vi "ziExample-UHFLI-Module-AWG.vi"() -> ()   [LabVIEW 2009]
doc: "Control a Zurich instrument device via the LabOne Labview API. \nRequirements: Zurich Instruments UHFLI \nThis example shows how to start a AWG module and measure it with the scope module.\n\n© Zurich Instruments AG, www.zhinst.com"
uses:
  <instrlib>/Zurich Instruments LabOne/Public/Modules/ziTypeModEnum.ctl
  <instrlib>/Zurich Instruments LabOne/Public/Configure/ziSetValueDouble.vi
  <instrlib>/Zurich Instruments LabOne/Public/Configure/ziSetValueDoubleArray.vi
  <instrlib>/Zurich Instruments LabOne/Public/Modules/ziModSetValueBinary.vi
  <instrlib>/Zurich Instruments LabOne/Public/Modules/ziModSetValueDoubleArray.vi
  <instrlib>/Zurich Instruments LabOne/Public/Modules/ziModGetScopeWave.vi
  <instrlib>/Zurich Instruments LabOne/Zurich Instruments LabOne.lvlib
panel:
  out "Status":bool
  out "Finish":bool
  out "Scopeready":bool caption="scopeready"
  out "?":cluster{dbl[], "Data Float":sgl[]}[](graph)
  in  "AWG":string="// Define an integer constant\nconst N = 4096;\n// Create  Gaussian pulses with length N points,\n// amplitude +1.0, center at N/2, and a width of N/8\nwave gauss = 1.0*gauss(N, N/2, N/8);\n\nplayWave(gauss);\nsetTrigger(1);\nsetTrigger(0);"
  out "Error Out":errorcluster
  in  "Address":string="DEV"
  out "Selected Device":string
  # "ziExample-UHFLI-Module-AWGvi\nRequirements: UHFLI\nsee block diagram for VI description"
  # "Tested Devices:\n- UHFLI"
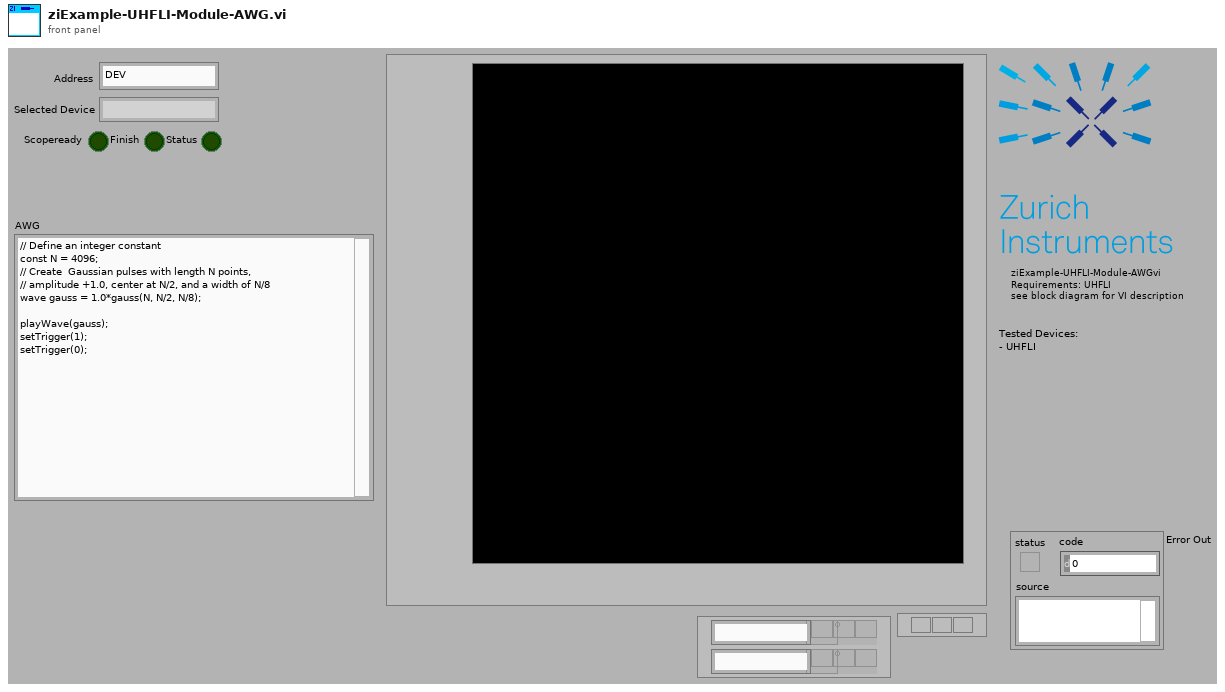
[diagram p1: front panel]
types:
  T1 = typedef "Zurich Instruments LabOne.lvlib/ziTypeModEnum.ctl" = u16
  T2 = typedef "Zurich Instruments LabOne.lvlib/ziTypeHandle.ctl" = cluster{"handleValid":bool, "Conn":u64, "Path Prefix":string, "Handle":u64, "Connected":bool, "Clockbase(s)":dbl}
  T3 = typedef "Zurich Instruments LabOne.lvlib/ziTypeModHandle.ctl" = cluster{"handleValid":bool, "Conn":u64, "ModHandle":u64, "moduleID":string, "Path Prefix":string}
  T4 = typedef "Zurich Instruments LabOne.lvlib/ziTypeModResults.ctl" = cluster{"PathArray":string[], "ValueType":T5, "NoOfResults":u64, "ziGenericHeader":T6[]}
  T5 = typedef "Zurich Instruments LabOne.lvlib/ziTypePollType.ctl" = enum16{"NONE", "DOUBLE_DATA", "INTEGER_DATA", "DEMOD_SAMPLE", "SCOPE_WAVE_HF2", "AUXIN_SAMPLE", "DIO_SAMPLE", "BYTE_ARRAY", "PWA_WAVE", "9", "10", "11", "12", "13", "14", "15", "TREE_CHANGE_DEPRI", "17", "ERROR", "19", "20", "21", "22", "23", "24", "25", "26", "27", "28", "29", "30", "31", "DOUBLE_DATA_TS", "INTEGER_DATA_TS", "34", "SCOPE_WAVE", "SCOPE_WAVE_EX", "37", "BYTE_ARRAY_TS", "39", "40", "41", "42", "43", "44", "45", "CNT_DATA", "47", "TREE_CHANGE", "49", "50", "51", "52", "53", "54", "55", "56", "57", "58", "59", "60", "61", "62", "63", "SWEEPER_DATA", "SPECTRUM_DATA", "ADVISOR_DATA", "VECTOR_DATA", "IMP_DATA", "SHF_GENERATOR_WAVEFORM_DATA", "SHF_RESULT_LOGGER_DATA", "SHF_SCOPE_DATA", "DEMOD_VECTOR"}
  T6 = typedef "Zurich Instruments LabOne.lvlib/ziTypeModGenericHeader.ctl" = cluster{"HeaderType":enum8{"HEADER_TYPE_NONE", "HEADER_TYPE_SWTRIGGER", "HEADER_TYPE_SWEEPER"}, "SampleFormat":u8, "SystemTime":timestamp, "CreatedTimeStamp":u64, "ChangedTimeStamp":u64, "Flags":u32, "ChunkSizeBytes":u64, "Name":string, "Status":u32, "GroupIndex":u32, "Color":u32, "ActiveRow":u32, "TriggerNumber":u64, "GridRows":u32, "GridCols":u32, "GridMode":u32, "GridOperation":u32, "GridDirection":u32, "GridRepetitions":u32, "GridColDelta":dbl, "GridColOffset":dbl, "GridRowDelta":dbl, "GridRowOffset":dbl, "Bandwidth":dbl, "Center":dbl, "Nenbw":dbl}
  T7 = typedef "Zurich Instruments LabOne.lvlib/ziTypeScopeWave.ctl" = cluster{"Timestamp (ticks)":u64, "Timestamp Trigger (ticks)":u64, "dt (s)":dbl, "Channel Enable":u8[], "Channel Input":enum8{"Signal Input 1", "Signal Input 2", "Trigger Input 1", "Trigger Input 2", "Aux Output 1", "Aux Output 2", "Aux Output 3", "Aux Output 4", "Aux Input 1", "Aux Input 2"}[], "Trigger Enable":u64, "Trigger Input":u64, "Channel BW Limit":u8[], "Channel Math":u8[], "Channel Scaling":sgl[], "Sequence Number":u32, "Segment Number":u32, "Block Number":u32, "Data Transfer Mode":enum8{"Single Transfer", "Block Transfer", "Continuous Transfer", "FFT Single Transfer"}, "Block Marker":enum8{"None", "End of Block"}, "Flags":u8, "Sample Format":enum8{"Int16", "Int32", "Float32", "reserved", "Int16 Interleaved", "Int32 Interleaved", "Float32 Interleaved"}, "Sample Count":u32, "Channel Offset":dbl[], "Data Int16":i16[], "Data Int32":i32[], "Data Float":sgl[], "Total Samples":u64}
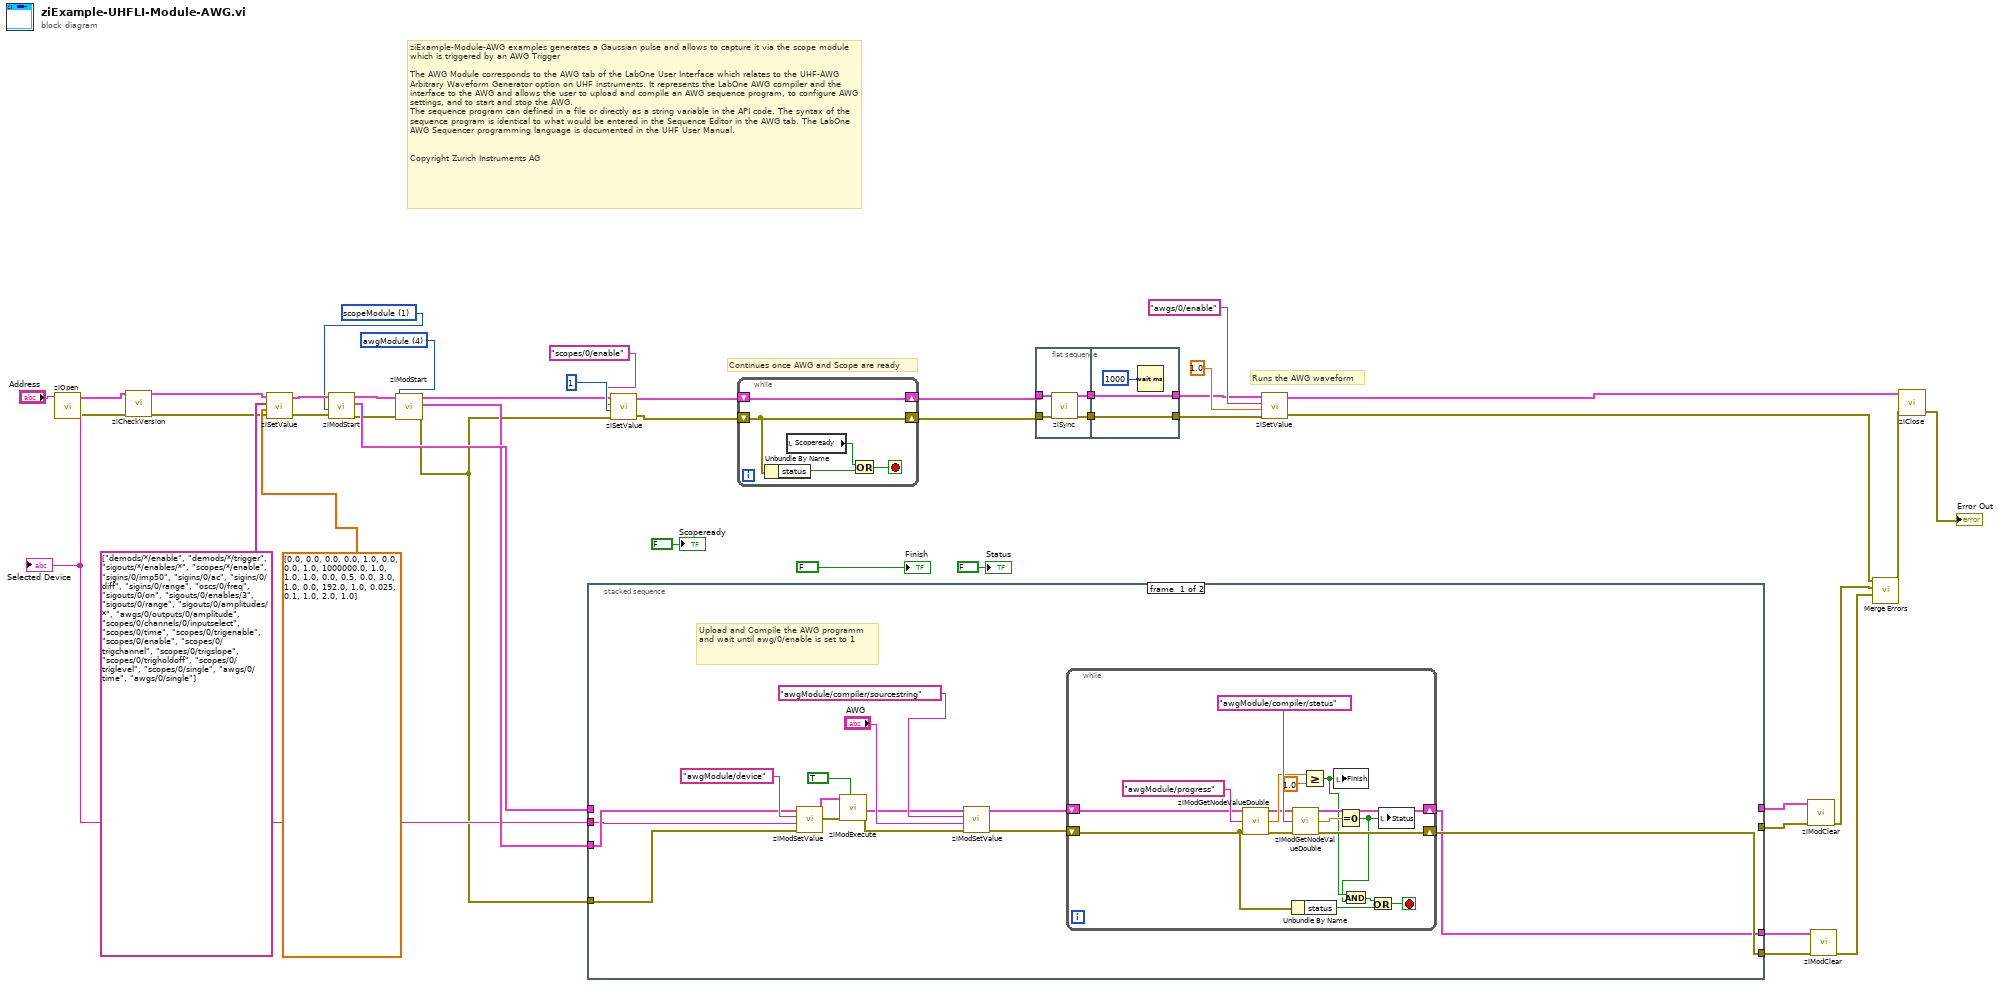
[diagram p0: block diagram]
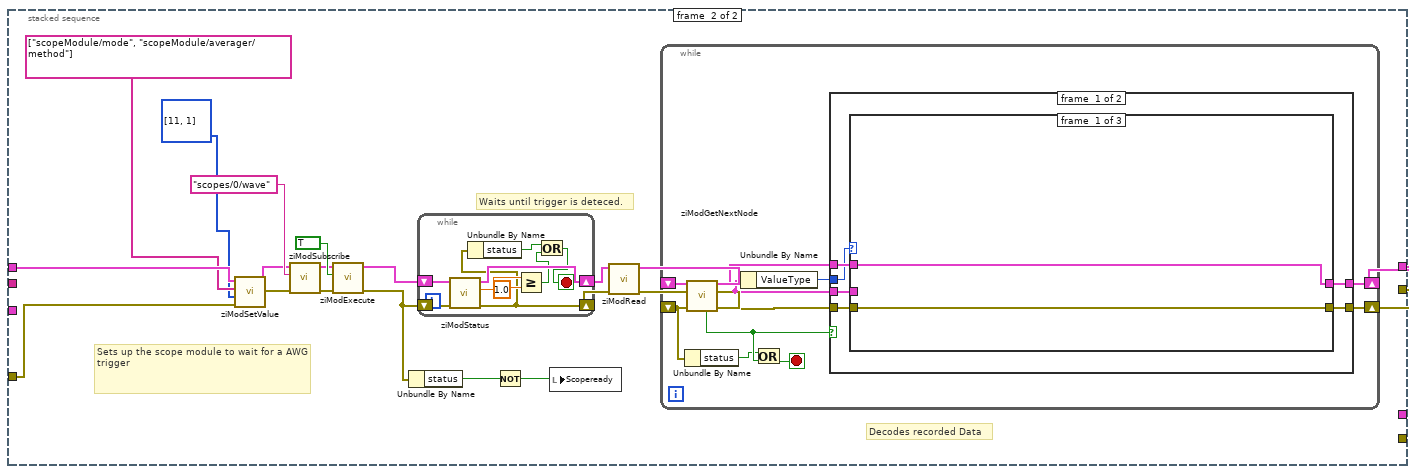
[diagram p2: hidden frame]
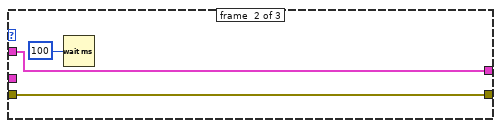
[diagram p3: hidden frame]
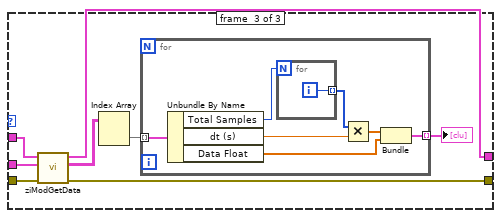
[diagram p4: hidden frame]
diagram:
  w6 = T1 4 items=["sweep", "scopeModule", "dataAcquisitionModule", "pidAdvisor", "awgModule", "impedanceModule", "multiDeviceSyncModule", "zoomFFT", "trigger", "deviceSettings", "record"] ("module Id")
  w5 = T1 1 items=["sweep", "scopeModule", "dataAcquisitionModule", "pidAdvisor", "awgModule", "impedanceModule", "multiDeviceSyncModule", "zoomFFT", "trigger", "deviceSettings", "record"] ("module Id")
  # "Runs the AWG waveform"
  # "Continues once AWG and Scope are ready"
  # "ziExample-Module-AWG examples generates a Gaussian pulse and allows to capture it via the scope module which is triggered by an AWG Trigger\n\nThe AWG Module corresponds to the AWG tab of the LabOne User Interface which relates to the UHF-AWG Arbitrary Waveform Generator option on UHF instruments. It represents the LabOne AWG compiler and the interface to the AWG and allows the user to upload and compile an AWG sequence program, to configure AWG settings, and to start and stop the AWG.\nThe sequence program can defined in a file or directly as a string variable in the API code. The syntax of the sequence program is identical to what would be entered in the Sequence Editor in the AWG tab. The LabOne AWG Sequencer programming language is documented in the UHF User Manual.\n\n\nCopyright Zurich Instruments AG"
  n1 = call <instrlib>:"ziOpen.vi"("Address"="Address") -> ("Error Out"=w10:errorcluster, "Selected Device"=w27:string, "HandleOut"=w7:T2)  [unwired: 1 in, 2 out]
  "Selected Device" <- w27
  n2 = call <instrlib>:"ziCheckVersion.vi"("Handle In"=w7, "Error In"=w10) -> ("Handle Out"=w8:T2, "Error Out"=w9:errorcluster)  [unwired: 11 in, 1 out]
  n3 = call-poly <instrlib>:"ziSetValue.vi"("Error In"=w9, "Values"=dbl[] [0.0, 0.0, 0.0, 0.0, 1.0, 0.0, 0.0, 1.0, 1000000.0, 1.0, 1.0, 1.0, 0.0, 0.5, 0.0, 3.0, 1.0, 0.0, 192.0, 1.0, 0.025, 0.1, 1.0, 2.0, 1.0], "Paths"=string[] ["demods/*/enable", "demods/*/trigger", "sigouts/*/enables/*", "scopes/*/enable", "sigins/0/imp50", "sigins/0/ac", "sigins/0/diff", "sigins/0/range", "oscs/0/freq", "sigouts/0/on", "sigouts/0/enables/3", "sigouts/0/range", "sigouts/0/amplitudes/*", "awgs/0/outputs/0/amplitude", "scopes/0/channels/0/inputselect", "scopes/0/time", "scopes/0/trigenable", "scopes/0/enable", "scopes/0/trigchannel", "scopes/0/trigslope", "scopes/0/trigholdoff", "scopes/0/triglevel", "scopes/0/single", "awgs/0/time", "awgs/0/single"], "Handle In"=w8) -> ("Error Out"=w29:errorcluster, "Handle Out"=w33:T2)  [unwired: 1 in]
  n4 = call <instrlib>:"ziModStart.vi"("Error In"=w29, "module Id"=w5, "Handle In"=w33) -> ("Error Out"=w28:errorcluster, "ModHandle Out"=w31:T3, "Handle Out"=w32:T2)  [unwired: 6 in]
  n5 = call <instrlib>:"ziModStart.vi"("Error In"=w28, "module Id"=w6, "Handle In"=w32) -> ("Error Out"=w12:errorcluster, "ModHandle Out"=w30:T3, "Handle Out"=w11:T2)  [unwired: 6 in]
  n6 = stacked-sequence {
    tunnel: w31 -> [_ w81]
    tunnel: [w54 _] -> w35
    tunnel: [w53 _] -> w36
    tunnel: [_ w83] -> w34
    tunnel: [_ w82] -> w37
    tunnel: w30 -> [w52 _]
    tunnel: w12 -> [w51 w80]
    tunnel: w27 -> [w50 _]
    frame #0 {
      # "Upload and Compile the AWG programm and wait until awg/0/enable is set to 1"
      n7 = call-poly <instrlib>:"ziModSetValue.vi"("Error In"=w51, "Data"=w50, "Path"="awgModule/device", "ModHandle In"=w52) -> ("Error Out"=w58:errorcluster, "ModHandle Out"=w57:T3)  [unwired: 6 in]
      n8 = call <instrlib>:"ziModExecute.vi"("Error In"=w58, "Modal (F)"=TRUE, "ziModHandle In"=w57) -> ("Error Out"=w46:errorcluster, "ziModHandle Out"=w47:T3)  [unwired: 6 in]
      n9 = call-poly <instrlib>:"ziModSetValue.vi"("Error In"=w46, "Data"="AWG", "Path"="awgModule/compiler/sourcestring", "ModHandle In"=w47) -> ("Error Out"=w44:errorcluster, "ModHandle Out"=w45:T3)  [unwired: 6 in]
      n10 = while {
        shift-right: [w67] -> w53
        shift-left: w45 -> [w69]
        shift-right: [w66] -> w54
        shift-left: w44 -> [w62]
        stop <- w64 stop-if-true
        n11 = call <instrlib>:"ziModGetNodeValueDouble.vi"("ModHandle In"=w69, "Path"="awgModule/progress", "error in"=w62) -> ("ModHandle Out"=w68:T3, "Value"=w71:dbl, "error out"=w65:errorcluster)  [unwired: 10 in]
        n12 = Unbundle By Name(w62) -> ("status"=w61:bool)
        n13 = call <instrlib>:"ziModGetNodeValueDouble.vi"("ModHandle In"=w68, "Path"="awgModule/compiler/status", "error in"=w65) -> ("ModHandle Out"=w67:T3, "Value"=w70:dbl, "error out"=w66:errorcluster)  [unwired: 10 in]
        n14 = Greater Or Equal?(x=w71, y=1.0) -> (x >= y?=w60:bool)
        n15 = local write "Finish"(w60) -> ()
        n16 = Equal To 0?(x=w70) -> (x = 0?=w59:bool)
        n17 = And(x=w60, y=w59) -> (x .and. y?=w63:bool)
        n18 = Or(x=w63, y=w61) -> (x .or. y?=w64:bool)
        n19 = local write "Status"(w59) -> ()
      }
    }
    frame #1 {
      # "Decodes recorded Data"
      # "Waits until trigger is deteced."
      # "Sets up the scope module to wait for a AWG trigger"
      n20 = call-poly <instrlib>:"ziModSetValue.vi"("Error In"=w80, "Values"=i32[] [11, 1], "Paths"=string[] ["scopeModule/mode", "scopeModule/averager/method"], "ModHandle In"=w81) -> ("Error Out"=w87:errorcluster, "ModHandle Out"=w88:T3)  [unwired: 6 in]
      n21 = call <instrlib>:"ziModSubscribe.vi"("Error In"=w87, "Path"="scopes/0/wave", "ModHandle In"=w88) -> ("Error Out"=w85:errorcluster, "ModHandle Out"=w86:T3)  [unwired: 6 in]
      n22 = call <instrlib>:"ziModExecute.vi"("Error In"=w85, "Modal (F)"=TRUE ("Modal"), "ziModHandle In"=w86) -> ("Error Out"=w79:errorcluster, "ziModHandle Out"=w84:T3)  [unwired: 6 in]
      n23 = Unbundle By Name(w79) -> ("status"=w78:bool)
      n24 = while {
        shift-right: [w99] -> w92
        shift-left: w84 -> [w103]
        shift-right: [w95] -> w91
        shift-left: w79 -> [w102]
        stop <- w96 stop-if-true
        n25 = call <instrlib>:"ziModStatus.vi"("Error In"=w102, "ModHandle IN"=w103) -> ("Error Out"=w95:errorcluster, "Progress (unity)"=w101:dbl, "ModHandle Out"=w99:T3)  [unwired: 5 in, 1 out]
        n26 = Unbundle By Name(w95) -> ("status"=w98:bool)
        n27 = Greater Or Equal?(x=w101, y=1.0) -> (x >= y?=w97:bool)
        n28 = Or(x=w98, y=w97) -> (x .or. y?=w96:bool)
      }
      n29 = Not(x=w78) -> (.not. x?=w75:bool)
      n30 = local write "Scopeready"(w75) -> ()
      n31 = call <instrlib>:"ziModRead.vi"("error in"=w91, "ziModHandle In"=w92) -> ("error out"=w94:errorcluster, "ziModHandle Out"=w93:T3)  [unwired: 8 in]
      n32 = while {
        shift-right: [w113] -> w82
        shift-left: w93 -> [w108]
        shift-right: [w112] -> w83
        shift-left: w94 -> [w104]
        stop <- w107 stop-if-true
        n33 = Unbundle By Name(w104) -> ("status"=w105:bool)
        n34 = call <instrlib>:"ziModGetNextNode.vi"("Error In"=w104, "ModHandle In"=w108) -> ("Error Out"=w111:errorcluster, "ModResults"=w109:T4, "ModHandle Out"=w114:T3, "NoData"=w106:bool)  [unwired: 6 in]
        n35 = Unbundle By Name(w109) -> ("ValueType"=w110:T5)
        n36 = Or(x=w105, y=w106) -> (x .or. y?=w107:bool)
        n37 = case shown="False" w106 {
          tunnel: w114 -> [w120 w142]
          tunnel: [w119 w142] -> w113
          tunnel: [w118 w143] -> w112
          tunnel: w111 -> [w117 w143]
          tunnel: w109 -> [w116 _]
          tunnel: w110 -> [w115 _]
          frame #0 {
            n38 = case shown="\"SCOPE_WAVE_EX\"" w115 {
              tunnel: w120 -> [w122 w125 w130]
              tunnel: w116 -> [_ _ w133]
              tunnel: w117 -> [w121 w124 w132]
              tunnel: [w121 w124 w131] -> w118
              tunnel: [w122 w125 w129] -> w119
              frame #0 {
              }
              frame #1 {
                n39 = Wait (ms)(milliseconds to wait=u32 100) -> ()  [unwired: 1 out]
              }
              frame #2 {
                n40 = call-poly <instrlib>:"ziModGetData.vi"("Error In"=w132, "ModResults"=w133, "ModHandle In"=w130) -> ("Error Out"=w131:errorcluster, "ModScopeWave"=w127:T7[][], "ModHandle Out"=w129:T3)  [unwired: 5 in, 1 out]
                n41 = Index Array(array=w127) -> (element=w126:T7[])  [unwired: 2 in]
                n42 = for {
                  tunnel: w126 -> [w140] mode=indexing
                  tunnel: [w139] -> w128 mode=indexing
                  n43 = Unbundle By Name(w140) -> ("Total Samples"=w136:u64, "dt (s)"=w137:dbl, "Data Float"=w138:sgl[])
                  n44 = for {
                    N: w136 -> [_]
                    tunnel: [w141] -> w134 mode=indexing
                    i -> [w141]
                  }
                  n45 = Multiply(x=w134, y=w137) -> (x*y=w135:dbl[])
                  n46 = Bundle(w135, "Data Float"=w138) -> (w139:cluster{dbl[], "Data Float":sgl[]})  [unwired: 1 in]
                }
                "?" <- w128
              }
            }
          }
          frame #1 {
          }
        }
      }
    }
  }
  n47 = call-poly <instrlib>:"ziSetValue.vi"("Error In"=w12, "Value"=1, "Path"="scopes/0/enable", "Handle In"=w11) -> ("Error Out"=w13:errorcluster, "Handle Out"=w14:T2)  [unwired: 1 in]
  n48 = while {
    shift-right: [w147] -> w3
    shift-left: w13 -> [w147]
    shift-right: [w148] -> w4
    shift-left: w14 -> [w148]
    stop <- w144 stop-if-true
    n49 = Unbundle By Name(w147) -> ("status"=w146:bool)
    n50 = local read "Scopeready"() -> (w145:bool)
    n51 = Or(x=w145, y=w146) -> (x .or. y?=w144:bool)
  }
  n52 = flat-sequence {
    tunnel: w3 -> [w152]
    tunnel: w4 -> [w149]
    tunnel: [w151] -> w2
    tunnel: [w150] -> w1
    tunnel: [w154] -> w21
    tunnel: [w155] -> w22
    tunnel: w2 -> [w155]
    tunnel: w1 -> [w154]
    frame #0 {
      n53 = call <instrlib>:"ziSync.vi"("Handle In"=w149, "Error In"=w152) -> ("Handle Out"=w150:T2, "Error Out"=w151:errorcluster)  [unwired: 12 in]
    }
    frame #1 {
      n54 = Wait (ms)(milliseconds to wait=u32 1000) -> ()  [unwired: 1 out]
    }
  }
  n55 = call-poly <instrlib>:"ziSetValue.vi"("Error In"=w22, "Value"=1.0, "Path"="awgs/0/enable", "Handle In"=w21) -> ("Error Out"=w17:errorcluster, "Handle Out"=w39:T2)  [unwired: 1 in]
  n56 = call <instrlib>:"ziModClear.vi"("Error In"=w34, "ziModHandle In"=w37) -> ("Error Out"=w25:errorcluster)  [unwired: 7 in, 1 out]
  n57 = call <instrlib>:"ziModClear.vi"("Error In"=w35, "ziModHandle In"=w36) -> ("Error Out"=w26:errorcluster)  [unwired: 7 in, 1 out]
  n58 = call <vilib>:"Merge Errors.vi"("error in 3 (no error)"=w26, "error in 2 (no error)"=w25, "error in 1 (no error)"=w17) -> ("error out"=w38:errorcluster)  [unwired: 4 in]
  n59 = call <instrlib>:"ziClose.vi"("Error In"=w38, "Handle In"=w39) -> ("Error Out"=→"Error Out":errorcluster)  [unwired: 2 in, 1 out]
  "Finish" <- FALSE ("Finish")
  "Status" <- FALSE ("Status")
  "Scopeready" <- FALSE ("scopeready")
